vi "NextPow2.vi"(11 "x":dbl) -> (3 "2^x":dbl)   [LabVIEW 2018]
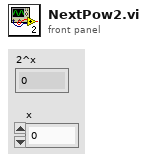
[diagram p1: front panel]
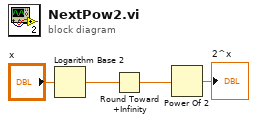
[diagram p0: block diagram]
diagram:
  n1 = Logarithm Base 2(1:"x") -> (0:w4:dbl)
  n2 = Round Toward +Infinity(x=w4) -> (ceil(x): smallest int >= x=w3:dbl)
  n3 = Power Of 2(x=w3) -> (2^x=→"2^x":dbl)
